vi "NI VeriStand - Undeploy UDP Channel Streaming Session.vi"(8 "error in (no error)":errorcluster, 11 "UDPChannelStreamSession in":T1) -> (0 "error out":errorcluster, 3 "UDPChannelStreamSession out":T1)   [LabVIEW 2020, in "NI_VS Workspace ExecutionAPI.lvlib"]
doc: "Undeploys a UDP channel streaming session and instructs the VeriStand Gateway to stop publishing UDP data."
uses:
  <vilib>/NI VeriStand/Execution/Workspace/NI_VS Workspace ExecutionAPI.lvlib
  <vilib>/NI VeriStand/Execution/Workspace/UDPChannelStreamSession.ctl
  NationalInstruments.VeriStand.ClientAPI
  NationalInstruments.VeriStand
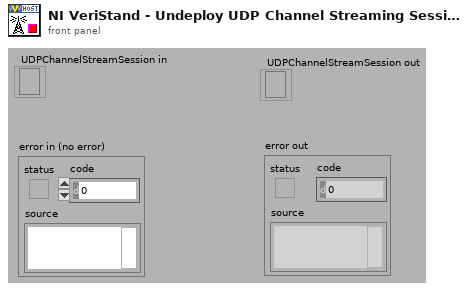
[diagram p1: front panel]
types:
  T1 = typedef "NI_VS Workspace ExecutionAPI.lvlib/UDPChannelStreamSession.ctl" = refnum<k24>
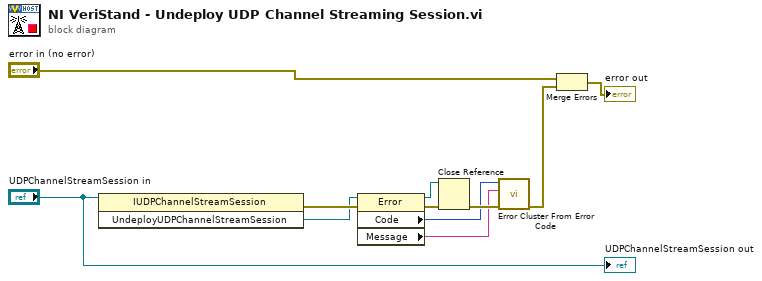
[diagram p0: block diagram]
diagram:
  n1 = invoke class="IUDPChannelStreamSession" method="UndeployUDPChannelStreamSession"(reference="UDPChannelStreamSession in") -> (error out=w10:errorcluster, "UndeployUDPChannelStreamSession"=w8:refnum<k24>)  [unwired: 2 in, 1 out]
  n2 = property class="Error"(reference=w8, error in=w10) -> (reference out=w7:refnum<k24>, error out=w9:errorcluster, "Code"=w5:u32, "Message"=w4:string)
  n3 = Close Reference(reference=w7, error in (no error)=w9) -> (error out=w6:errorcluster)
  n4 = call <vilib>:"Error Cluster From Error Code.vi"("error in (no error)"=w6, "error message (\"\")"=w4, "error code (0)"=w5) -> ("error out"=w11:errorcluster)  [unwired: 6 in]
  n5 = Merge Errors("error in (no error)", w11) -> (→"error out":errorcluster)
  "UDPChannelStreamSession out" <- "UDPChannelStreamSession in"
